vi "Write Standard.vi"(8 "error in (no error)":errorcluster, 10 "Standard":string, 11 "Servo MSMT in":refnum<class "Servo MSMT.lvclass">) -> (0 "error out":errorcluster, 3 "Servo MSMT out":refnum<class "Servo MSMT.lvclass">)   [LabVIEW 2018, in "Servo MSMT.lvlib" / "Servo MSMT.lvclass"]
uses:
  Servo MSMT.lvclass
  Servo MSMT.lvclass/Servo MSMT.ctl
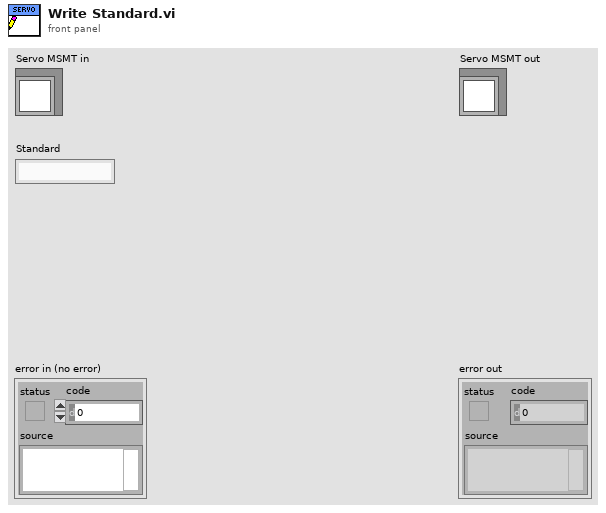
[diagram p1: front panel]
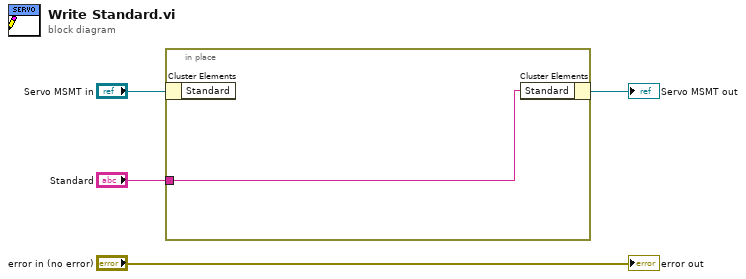
[diagram p0: block diagram]
diagram:
  n1 = in-place {
    in-place-border: "Standard" -> [w5]
    n2 = in-place-cluster #1("Servo MSMT in") -> ()  [unwired: 1 out]
    n3 = in-place-cluster #1("Standard"=w5) -> (→"Servo MSMT out":refnum<class "Servo MSMT.lvclass">)
  }
  "error out" <- "error in (no error)"
